vi "NI VeriStand - Add Custom Device Waveform.vi"(4 "Property Values":variant[](array[variant]), 5 "Highlight? (F)":bool, 6 "Property names":string[](array[string]), 7 "GUID (Default Waveform)":string="83F792DC-AED3-09DF-CB38-512C04DA274D", 8 "error in (no error)":errorcluster, 9 "Waveform":T2, 10 "Waveform Name":string, 11 "Parent Ref in":T1 format="%.0x") -> (0 "error out":errorcluster, 1 "Waveform Ref":T1 format="%.0x", 2 "Newly Created?":bool, 3 "Parent Ref out":T1 format="%.0x")   [LabVIEW 2026, in "Custom Devices Storage.lvlib"]
uses:
  Custom Devices Storage.lvlib
  <vilib>/NI VeriStand/Custom Device API/Custom Device Item Ref.ctl
  <vilib>/NI VeriStand/Custom Device API/Custom Device Waveform.ctl
  <vilib>/NI VeriStand/Custom Device API/Custom Device Waveform DataType.ctl
  C:/Users/Administrator/Desktop/Jatin/All DNC DLLs/NationalInstruments.VeriStand.SystemDefinitionAPI.dll
  Jatin/All DNC DLLs/NationalInstruments.VeriStand.SystemDefinitionAPI.dll
  <vilib>/NI VeriStand/Custom Device API/Custom Device API.lvlib
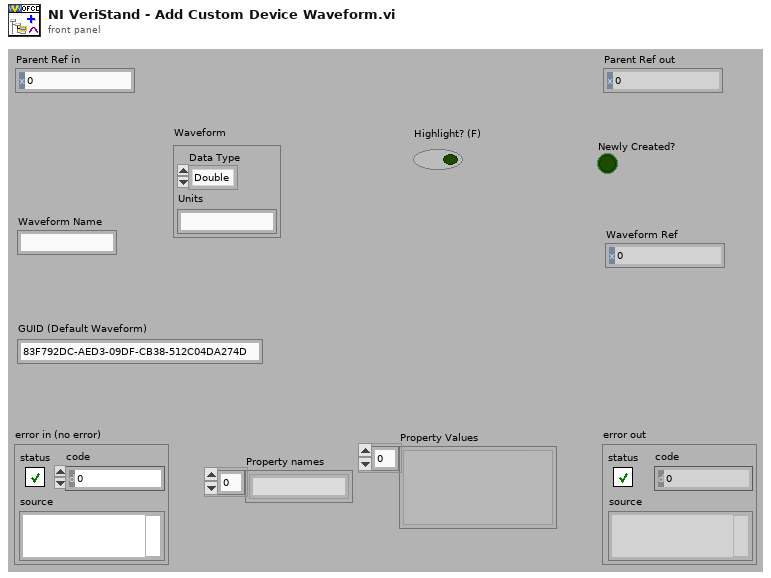
[diagram p1: front panel]
types:
  T1 = typedef "Custom Device API.lvlib/Custom Device Item Ref.ctl" = u64
  T2 = typedef "Custom Device API.lvlib/Custom Device Waveform.ctl" = cluster{"Data Type":T3, "Units":string}
  T3 = typedef "Custom Device API.lvlib/Custom Device Waveform DataType.ctl" = enum16{"Double", "Complex Double"}
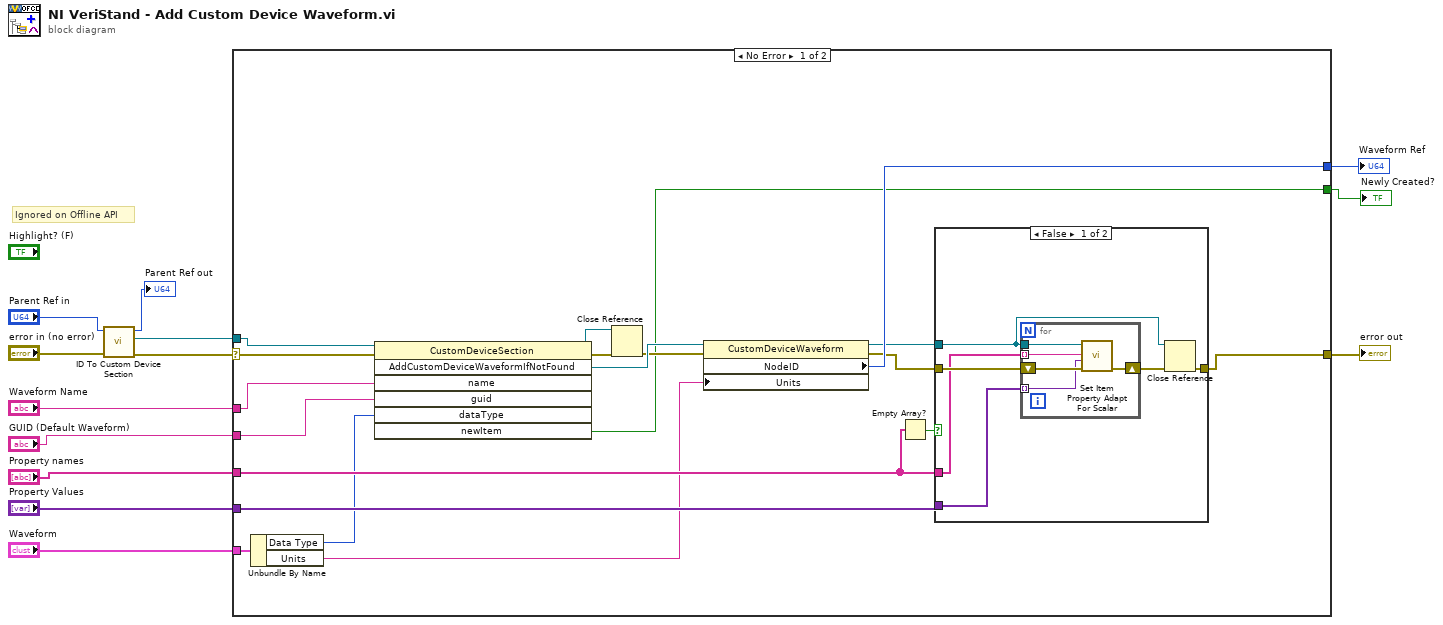
[diagram p0: block diagram]
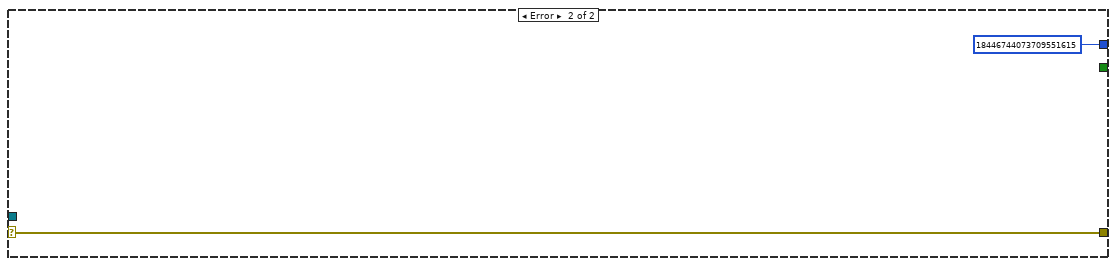
[diagram p3: hidden frame]
diagram:
  # "Ignored on Offline API"
  n1 = call "ID To Custom Device Section.vi"("error in (no error)"="error in (no error)", "ID in"="Parent Ref in") -> ("error out"=w13:errorcluster, "NationalInstruments.VeriStand.SystemDefinitionAPI.CustomDeviceSection"=w12:refnum<k39>, "ID out"=→"Parent Ref out":u64)  [unwired: 7 in]
  n2 = case shown="No Error" w13 {
    selector: w13 -> [w31 w46]
    tunnel: [w29 w46] -> w2
    tunnel: w12 -> [w32 _]
    tunnel: "GUID (Default Waveform)" -> [w30 _]
    tunnel: [w24 T1 18446744073709551615 ("Section Ptr")] -> w3
    tunnel: [w14 _] -> w4
    tunnel: "Property names" -> [w21 _]
    tunnel: "Property Values" -> [w20 _]
    tunnel: "Waveform Name" -> [w19 _]
    tunnel: "Waveform" -> [w18 _]
    frame No Error {
      n3 = Unbundle By Name(w18) -> ("Data Type"=w15:T3, "Units"=w17:string)
      n4 = invoke class="CustomDeviceSection" method="AddCustomDeviceWaveformIfNotFound"(reference=w32, error in=w31, "name"=w19, "guid"=w30, "dataType"=w15) -> (reference out=w27:refnum<k39>, error out=w28:errorcluster, "AddCustomDeviceWaveformIfNotFound"=w26:refnum<k39>, "newItem"=w14:bool)  [unwired: 2 in, 3 out]
      n5 = Close Reference(reference=w27, error in (no error)=w28) -> (error out=w25:errorcluster)
      n6 = property class="CustomDeviceWaveform"(reference=w26, error in=w25, "Units"=w17) -> (reference out=w22:refnum<k39>, error out=w23:errorcluster, "NodeID"=w24:u64)
      n7 = Empty Array?(array=w21) -> (empty?=w16:bool)
      n8 = case shown="False" w16 {
        tunnel: w22 -> [w34 _]
        tunnel: w23 -> [w38 w44]
        tunnel: w20 -> [w37 _]
        tunnel: w21 -> [w36 _]
        tunnel: [w33 w44] -> w29
        frame False {
          n9 = for {
            tunnel: w37 -> [w42] mode=indexing
            tunnel: w36 -> [w41] mode=indexing
            shift-right: [w39] -> w35
            shift-left: w38 -> [w43]
            tunnel: w34 -> [w40]
            n10 = call "Set Item Property Adapt For Scalar.vi"("error in (no error)"=w43, "Value"=w42, "Property Name"=w41, "NationalInstruments.VeriStand.SystemDefinitionAPI.CustomDeviceBase"=w40) -> ("error out"=w39:errorcluster)  [unwired: 5 in, 2 out]
          }
          n11 = Close Reference(reference=w34, error in (no error)=w35) -> (error out=w33:errorcluster)
        }
        frame True {
        }
      }
    }
    frame Error {
    }
  }
  "error out" <- w2
  "Waveform Ref" <- w3
  "Newly Created?" <- w4
